vi "Fetch Multi Eval Meas IEM Margin Power Results.vi"(8 "error in (no error)":errorcluster, 9 "Result Type (Current)":i32(ring) items=["Current"=0, "Extreme"=2], 10 "Instance (1)":T2=1, 11 "VISA resource name":refnum<visa-resource-name>) -> (0 "error out":errorcluster, 1 "Margin Power Results":T1 {"Carrier Leakage" format="%^.3e"; "IQ Image" format="%^.3e"; "General" format="%^.3e"; "Out Of Tolerance" format="%^.3e"}, 2 "Reliability":i32, 3 "VISA resource name out":refnum<visa-resource-name>)   [LabVIEW 2015, in "Rohde&Schwarz CMXP NR FR2 Measurement.lvlib"]
doc: "Returns the multi eval measurement IEM power limit line margin results.\n\nAttributes:\nRSCMXPNRFR2M_ATTR_FETCH_MULTI_EVAL_MEASUREMENT_IEM_MARGIN_CURRENT_POWER_RESULTS\nRSCMXPNRFR2M_ATTR_FETCH_MULTI_EVAL_MEASUREMENT_IEM_MARGIN_EXTREME_POWER_RESULTS\n\nRemote-control commands:\nFETCh:NRMMw:MEAS<i>:MEValuation:IEMission:MARGin:CURRent:POWer?\nFETCh:NRMMw:MEAS<i>:MEValuation:IEMission:MARGin:EXTReme:POWer?"
uses:
  <instrlib>/Rohde&Schwarz CMXP NR FR2 Measurement/Rohde&Schwarz CMXP NR FR2 Measurement.lvlib
  <instrlib>/Rohde&Schwarz CMXP NR FR2 Measurement/Private/_Instance.ctl
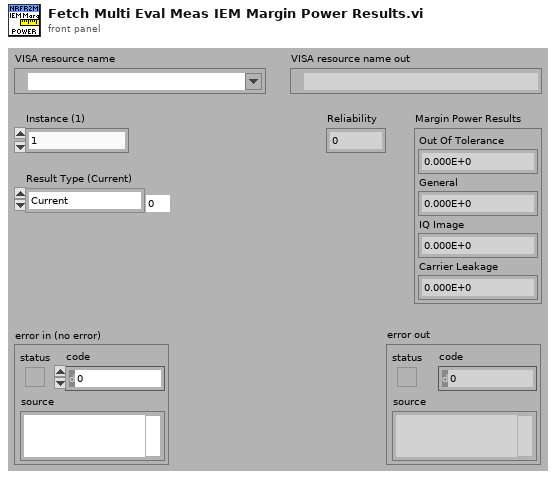
[diagram p1: front panel]
types:
  T1 = cluster{"Out Of Tolerance":dbl, "General":dbl, "IQ Image":dbl, "Carrier Leakage":dbl}
  T2 = typedef "Rohde&Schwarz CMXP NR FR2 Measurement.lvlib/_Instance.ctl" = i32
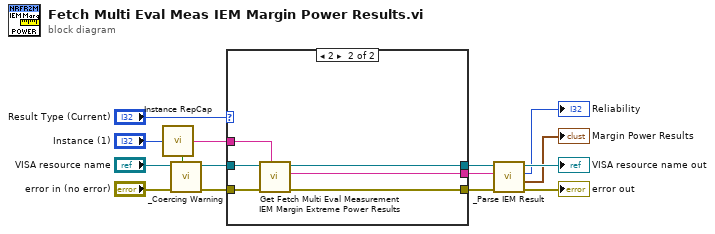
[diagram p0: block diagram]
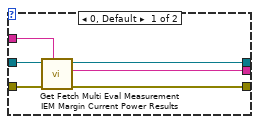
[diagram p2: hidden frame]
diagram:
  n1 = call <instrlib>:"Instance RepCap.vi"("Instance In"="Instance (1)") -> ("In Range?"=w4:bool, "RepCap Identifier Out"=w8:string)  [unwired: 1 in]
  n2 = call <instrlib>:"_Coercing Warning.vi"("In Range?"=w4, "error in (no error)"="error in (no error)", "VISA resource name"="VISA resource name") -> ("error out"=w2:errorcluster, "VISA resource name out"=w3:refnum<visa-resource-name>)  [unwired: 7 in]
  n3 = case shown="2" "Result Type (Current)" {
    tunnel: w2 -> [w21 w27]
    tunnel: w3 -> [w20 w26]
    tunnel: [w19 w25] -> w15
    tunnel: [w18 w24] -> w14
    tunnel: [w17 w23] -> w13
    tunnel: w8 -> [w16 w22]
    frame 0, Default {
      n4 = call "Get Fetch Multi Eval Measurement IEM Margin Current Power Results"("Repeated Capabilities"=w16, "error in (no error)"=w21, "instrument handle"=w20) -> ("error out"=w17:errorcluster, "Fetch Multi Eval Measurement IEM Margin Current Power Results"=w18:string, "instrument handle out"=w19:refnum<visa-resource-name>)  [unwired: 6 in]
    }
    frame 2 {
      n5 = call "Get Fetch Multi Eval Measurement IEM Margin Extreme Power Results"("Repeated Capabilities"=w22, "error in (no error)"=w27, "instrument handle"=w26) -> ("error out"=w23:errorcluster, "Fetch Multi Eval Measurement IEM Margin Extreme Power Results"=w24:string, "instrument handle out"=w25:refnum<visa-resource-name>)  [unwired: 6 in]
    }
  }
  n6 = call <instrlib>:"_Parse IEM Result.vi"("error in (no error)"=w13, "Input String"=w14, "VISA resource name"=w15) -> ("error out"=→"error out":errorcluster, "Result"=→"Margin Power Results":T1, "Reliability"=→"Reliability":i32, "VISA resource name out"=→"VISA resource name out":refnum<visa-resource-name>)  [unwired: 5 in]
